vi "Initialize_FIFOs.vi"() -> (0 "FIFO Array":refnum<queue>[][][](array[refnum]))   [LabVIEW 2015]
panel:
  out "FIFO Lengths":i32[](array[numeric])=[50000, 25000, 12500, 6250, 3125, 1562, 781]
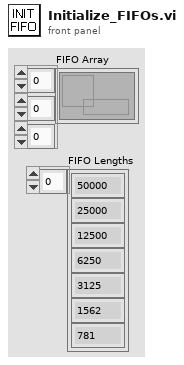
[diagram p1: front panel]
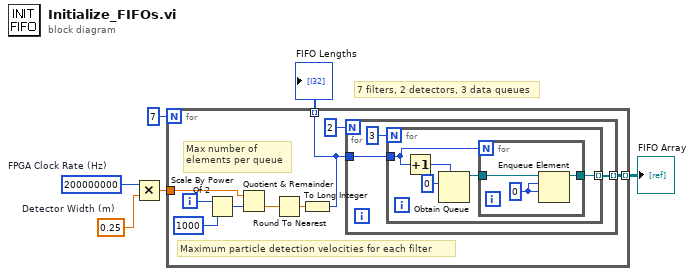
[diagram p0: block diagram]
diagram:
  w4 = sgl 0.25  # Detector Width (m)
  w5 = 200000000  # FPGA Clock Rate (Hz)
  # "7 filters, 2 detectors, 3 data queues"
  n1 = Multiply(x=w5, y=w4) -> (x*y=w3:sgl)
  n2 = for {
    N: 7 -> [_]
    tunnel: w3 -> [w12]
    tunnel: [w9] -> w2 mode=indexing
    tunnel: [w7] -> w1 mode=indexing
    i -> [w13]
    # "Max number of\nelements per queue"
    # "Maximum particle detection velocities for each filter"
    n3 = Scale By Power Of 2(n=w13, x=1000) -> (x*2^n=w11:i32)
    n4 = Quotient & Remainder(x=w12, y=w11) -> (floor(x/y)=w10:sgl)  [unwired: 1 out]
    n5 = Round To Nearest(number=w10) -> (nearest integer value=w8:sgl)
    n6 = To Long Integer(number=w8) -> (32bit integer=w7:i32)
    n7 = for {
      N: 2 -> [_]
      tunnel: [w17] -> w9 mode=indexing
      tunnel: w7 -> [w16]
      n8 = for {
        N: 3 -> [_]
        tunnel: [w19] -> w17 mode=indexing
        tunnel: w16 -> [w21]
        n9 = Increment(x=w21) -> (x+1=w20:i32)
        n10 = Obtain Queue(max queue size (-1, unlimited)=w20, element data type=0) -> (queue out=w22:refnum<queue>)  [unwired: 3 in, 2 out]
        n11 = for {
          N: w21 -> [_]
          tunnel: w22 -> [w26]
          tunnel: [w25] -> w19
          w24 = 0 ("element")
          n12 = Enqueue Element(queue=w26, element=w24, timeout in ms (-1)=w24) -> (queue out=w25:refnum<queue>)  [unwired: 1 in, 2 out]
        }
      }
    }
  }
  "FIFO Array" <- w2
  "FIFO Lengths" <- w1
